vi "SubVI - Get Connected SubVIs.vi"(8 "error in (no error)":errorcluster, 11 "SubVI in":refnum<vi>) -> (0 "error out":errorcluster, 3 "Array":refnum<vi>[](array[refnum]))   [LabVIEW 2017, in "csmHelper-SubVI.lvlib"]
uses:
  csmHelper-SubVI.lvlib
  Terminals/csmHelper-Terminals.lvlib
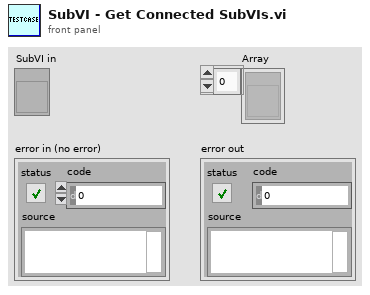
[diagram p1: front panel]
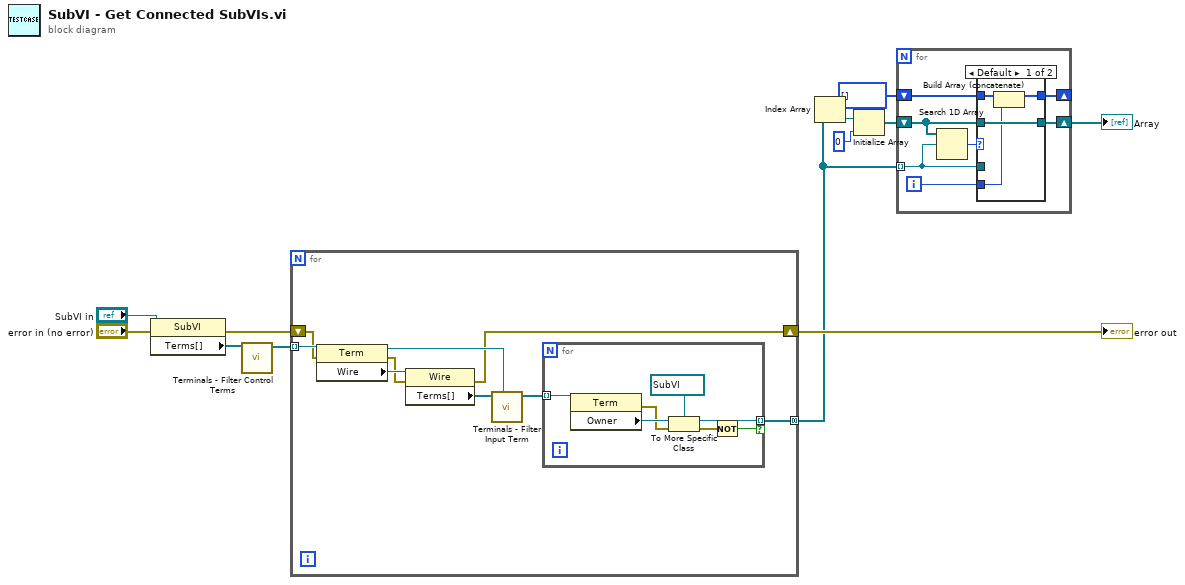
[diagram p0: block diagram]
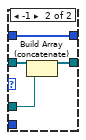
[diagram p2: hidden frame]
diagram:
  n1 = property on="Property Node" class="SubVI"(reference="SubVI in", error in="error in (no error)") -> (error out=w5:errorcluster, "Terms[]"=w3:refnum<vi>[])  [unwired: 1 out]
  n2 = call "Terminals - Filter Control Terms.vi"("Terms[]"=w3) -> ("Terms[] out"=w4:refnum<vi>[])  [unwired: 10 in]
  n3 = for {
    tunnel: w4 -> [w21] mode=indexing
    shift-right: [w14] -> w12
    shift-left: w5 -> [w15]
    tunnel: [w13] -> w10 mode=concatenating
    n4 = property class="Term"(reference=w21, error in=w15) -> (reference out=w18:refnum<vi>, error out=w16:errorcluster, "Wire"=w20:refnum<vi>)
    n5 = property class="Wire"(reference=w20, error in=w16) -> (error out=w14:errorcluster, "Terms[]"=w19:refnum<vi>[])  [unwired: 1 out]
    n6 = call "Terminals - Filter Input Term.vi"("InnerTerminal in"=w18, "Wire.Terms[] in"=w19) -> ("Wire.Terms[] out"=w17:refnum<vi>[])  [unwired: 9 in]
    n7 = for {
      tunnel: w17 -> [w28] mode=indexing
      tunnel: [w24] -> w13 mode=indexing if=w22
      n8 = property class="Term"(reference=w28) -> (error out=w25:errorcluster, "Owner"=w27:refnum<vi>)  [unwired: 1 in, 1 out]
      n9 = To More Specific Class(target class=refnum<vi> refnum ("reference out"), reference=w27, error in=w25) -> (specific class reference=w24:refnum<vi>, error out=w23:errorcluster)
      n10 = Not(x=w23) -> (.not. x?=w22:bool)
    }
  }
  "error out" <- w12
  n11 = Index Array(array=w10) -> (element=w7:refnum<vi>)  [unwired: 1 in]
  n12 = Initialize Array(w7, 0 ("Dimension Size")) -> (w8:refnum<vi>[])
  n13 = for {
    tunnel: w10 -> [w34] mode=indexing
    shift-right: [w33] -> w11
    shift-left: w8 -> [w32]
    shift-right: [w30] -> _
    shift-left: i32[] [] -> [w29]
    i -> [w31]
    n14 = Search 1D Array(1D array=w32, element=w34) -> (index of element=w35:i32)  [unwired: 1 in]
    n15 = case shown="Default" w35 {
      tunnel: w34 -> [_ w43]
      tunnel: [w39 w41] -> w33
      tunnel: w32 -> [w39 w42]
      tunnel: w31 -> [w36 _]
      tunnel: [w37 w40] -> w30
      tunnel: w29 -> [w38 w40]
      frame Default {
        n16 = Build Array (concatenate)(w38, w36) -> (w37:i32[])
      }
      frame -1 {
        n17 = Build Array (concatenate)(w42, w43) -> (w41:refnum<vi>[])
      }
    }
  }
  "Array" <- w11
